vi "Read Send Functionality.vi"(8 "error in (no error)":errorcluster, 11 "Instrument Msg in":refnum<class "Instrument Msg.lvclass">) -> (0 "error out":errorcluster, 1 "Timeout if Waiting":i32=-1, 2 "Send Function":T2=enum."Await Reply", 3 "Instrument Msg out":refnum<class "Instrument Msg.lvclass">, 4 "Message Priority":T1=enum."Normal", 5 "Publish Data?":bool=TRUE)   [LabVIEW 2020, in "Instrument Handler.lvlib" / "Instrument Msg.lvclass"]
doc: "Define the send functionality of the Instrument Msg."
uses:
  Instrument Msg.lvclass
  PPL/HDH.Actor Framework.Core.Publisher.lvlibp/Messages/Response Msg/Response Core/Controls/Ctl_SendFunction.ctl
  PPL/HDH.Actor Framework.Core.Actor.lvlibp/1abvi3w/vi.lib/ActorFramework/Message Enqueuer/Message Priority.ctl
  Instrument Msg.lvclass/Instrument Msg.ctl
  PPL/HDH.Actor Framework.Core.Publisher.lvlibp
  PPL/HDH.Actor Framework.Core.Actor.lvlibp/1abvi3w/vi.lib/ActorFramework/Message Enqueuer/Message Enqueuer.lvclass
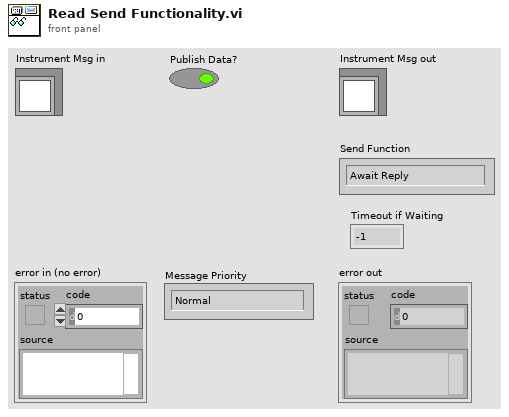
[diagram p1: front panel]
types:
  T1 = typedef "HDH.Actor Framework.Core.Actor.lvlibp/Message Enqueuer.lvclass/Message Priority.ctl" = enum16{"Low", "Normal", "High"}
  T2 = typedef "HDH.Actor Framework.Core.Publisher.lvlibp/Ctl_SendFunction.ctl" = enum16{"Send and Forget", "Request Reply", "Await Reply"}
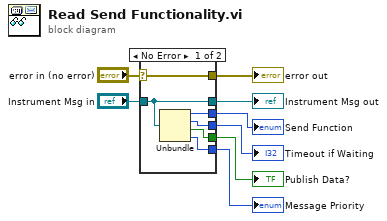
[diagram p0: block diagram]
diagram:
  n1 = case shown="No Error" "error in (no error)" {
    selector: "error in (no error)" -> [w14 w15]
    tunnel: [w14 w15] -> w7
    tunnel: [w10 w16] -> w5
    tunnel: "Instrument Msg in" -> [w10 w16]
    tunnel: [w13 _] -> w4
    tunnel: [w12 _] -> w3
    tunnel: [w11 _] -> w2
    tunnel: [w9 _] -> w1
    frame No Error {
      n2 = Unbundle(w10) -> (w13:T2, w11:i32, w12:bool, w9:u16)
    }
    frame Error {
    }
  }
  "error out" <- w7
  "Instrument Msg out" <- w5
  "Send Function" <- w4
  "Timeout if Waiting" <- w2
  "Publish Data?" <- w3
  "Message Priority" <- w1
